vi "GA_Single Breed.vi"(6 "Parameters":T2={"Population size"=0, "Generations no."=0, "Crossover probabality"=0.0, "Mutation mode"=enum."one-point, fixed rate", "Creep mutation"=FALSE, "Mutation rate"=0.005, "Min mutation rate"=0.0, "Max mutation rate"=0.0, "Relative fitness differential"=0.0, "Reproduction plan"=enum."Full generational replacement", "Elitism"=FALSE, "FeaturesPerChannel"=0} {"Relative fitness differential" min=0.0 max=1.0; "Max mutation rate" min=0.0 max=1.0; "Min mutation rate" min=0.0 max=1.0; "Mutation rate" min=0.0 max=1.0; "Crossover probabality" min=0.0 max=1.0; "Generations no." min=1; "Population size" min=1}, 11 "Population in":T1) -> (0 "Offsprings":i8[][](array[numeric]), 3 "Population out":T1)   [LabVIEW 2016, in "GA.lvlib"]
doc: "Selects two parents from population and creates two children"
uses:
  GA.lvlib
  GA_tParameters.ctl
  GA_tPopulation.ctl
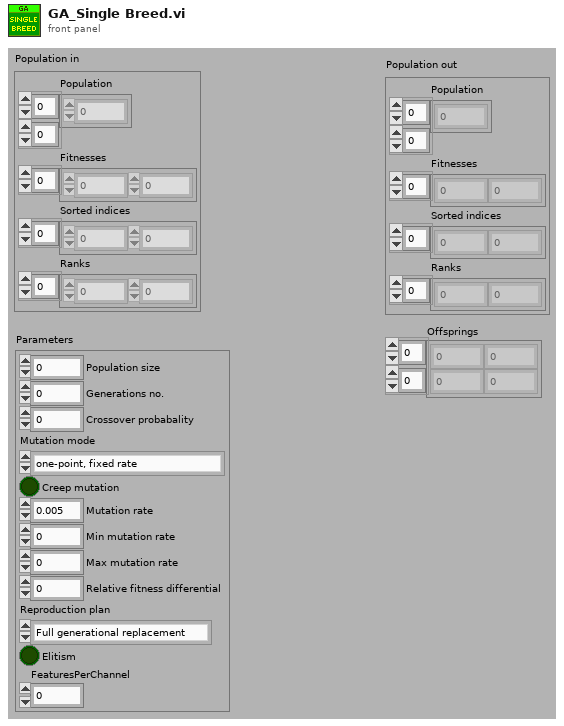
[diagram p1: front panel]
types:
  T1 = typedef "GA.lvlib/GA_tPopulation.ctl" = cluster{"Population":i8[][], "Fitnesses":dbl[], "Sorted indices":i32[], "Ranks":i32[]}
  T2 = typedef "GA.lvlib/GA_tParameters.ctl" = cluster{"Population size":i32, "Generations no.":i32, "Crossover probabality":dbl, "Mutation mode":enum16{"one-point, fixed rate", "one-point, fitness-adjustable rate", "one-point, distance-adjustable rate"}, "Creep mutation":bool, "Mutation rate":dbl, "Min mutation rate":dbl, "Max mutation rate":dbl, "Relative fitness differential":dbl, "Reproduction plan":enum16{"Full generational replacement", "Steady-state-replace-random", "Steady-state-replace-worst"}, "Elitism":bool, "FeaturesPerChannel":i32}
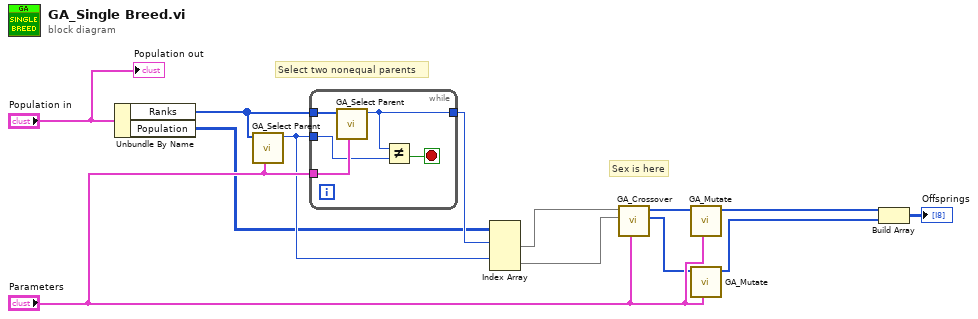
[diagram p0: block diagram]
diagram:
  # "Sex is here"
  # "Select two nonequal parents"
  n1 = Unbundle By Name("Population in") -> ("Ranks"=w7:i32[], "Population"=w6:i8[][])
  n2 = call "GA_Select Parent.vi"("Parameters"="Parameters", "Ranks"=w7) -> ("Parent index"=w10:i32)  [unwired: 9 in]
  n3 = while {
    tunnel: w10 -> [w16]
    tunnel: w7 -> [w18]
    tunnel: "Parameters" -> [w17]
    tunnel: [w14] -> w9
    stop <- w15 stop-if-true
    n4 = call "GA_Select Parent.vi"("Parameters"=w17, "Ranks"=w18) -> ("Parent index"=w14:i32)  [unwired: 9 in]
    n5 = Not Equal?(x=w14, y=w16) -> (x != y?=w15:bool)
  }
  n6 = Index Array(array=w6, index (row) #1=w9, index (row) #2=w10) -> (element #1=w5:i8[], element #2=w4:i8[])  [unwired: 2 in]
  n7 = call "GA_Crossover.vi"("Parameters"="Parameters", "Genotype 2"=w4, "Genotype 1"=w5) -> ("Offspring 2"=w11:i8[], "Offspring 1"=w12:i8[])  [unwired: 7 in]
  n8 = call "GA_Mutate.vi"("Parameters"="Parameters", "Genotype in"=w12) -> ("Genotype out"=w3:i8[])  [unwired: 9 in]
  n9 = call "GA_Mutate.vi"("Parameters"="Parameters", "Genotype in"=w11) -> ("Genotype out"=w2:i8[])  [unwired: 9 in]
  n10 = Build Array(w3, w2) -> (→"Offsprings":i8[][])
  "Population out" <- "Population in"
